vi "Find First Matching Resource (String).vi"(6 "Error if not found? (F)":bool, 8 "error in (no error)":errorcluster, 10 "Resource Types":string[](array[string]), 11 "Resources":T1) -> (0 "error out":errorcluster, 1 "Index":i32, 2 "Found?":bool, 3 "Resource":T2)   [LabVIEW 2023]
uses:
  CTLs/Resource.ctl
  CTLs/Resource Array.ctl
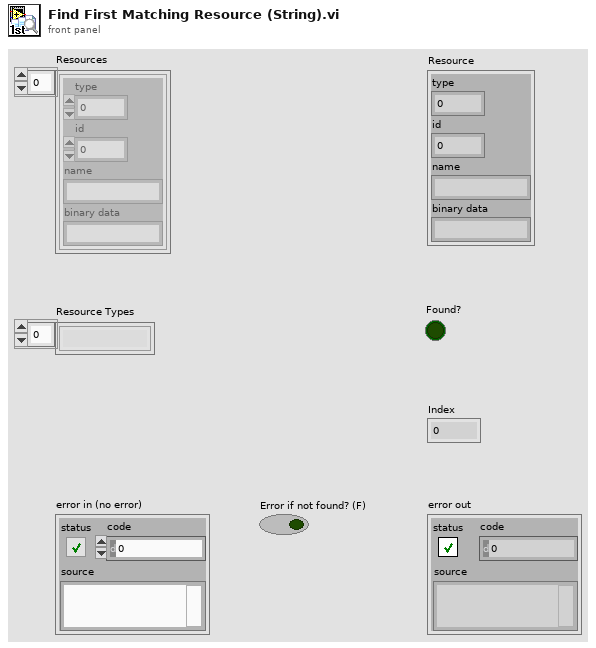
[diagram p1: front panel]
types:
  T1 = typedef "Resource Array.ctl" = T2[]
  T2 = typedef "Resource.ctl" = cluster{"type":u32, "id":i32, "name":string, "binary data":string}
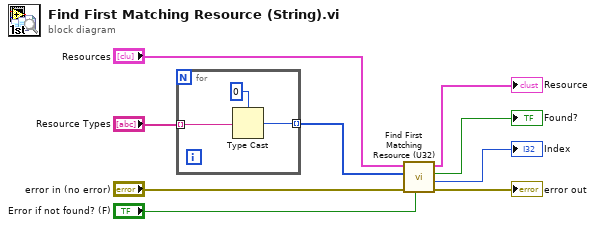
[diagram p0: block diagram]
diagram:
  n1 = for {
    tunnel: "Resource Types" -> [w11] mode=indexing
    tunnel: [w10] -> w7 mode=indexing
    n2 = Type Cast(type=u32 0, x=w11) -> (*(type *) &x=w10:u32)
  }
  n3 = call "Find First Matching Resource (U32).vi"("Error if not found? (F)"="Error if not found? (F)", "error in (no error)"="error in (no error)", "Resource Types"=w7, "Resources"="Resources") -> ("error out"=→"error out":errorcluster, "Index"=→"Index":i32, "Found?"=→"Found?":bool, "Resource"=→"Resource":T2)  [unwired: 4 in]
